vi "Update.vi"(10 "Value":dbl, 11 "OscillationDetector in":refnum<class "OscillationDetector.lvclass">) -> (3 "OscillationDetector out":refnum<class "OscillationDetector.lvclass">)   [LabVIEW 2019, in "OscillationDetector.lvclass"]
uses:
  OscillationDetector.lvclass
  OscillationDetector.lvclass/OscillationDetector.ctl
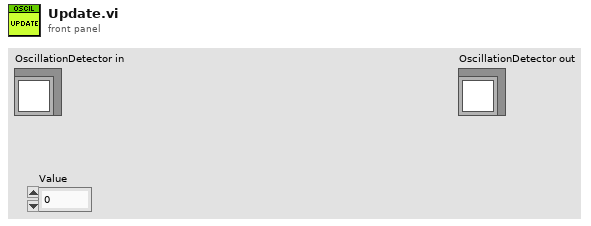
[diagram p1: front panel]
types:
  T1 = typedef "DATA Oscill.ctl" = cluster{"SUM":dbl, "COUNTER":dbl, "MAX CURR":dbl, "MIN CURR":dbl, "AVR":dbl, "MAX":dbl, "MIN":dbl, "DELTA AVR":dbl, "DELTA MAX":dbl, "DELTA MIN":dbl, "PERIOD":dbl}
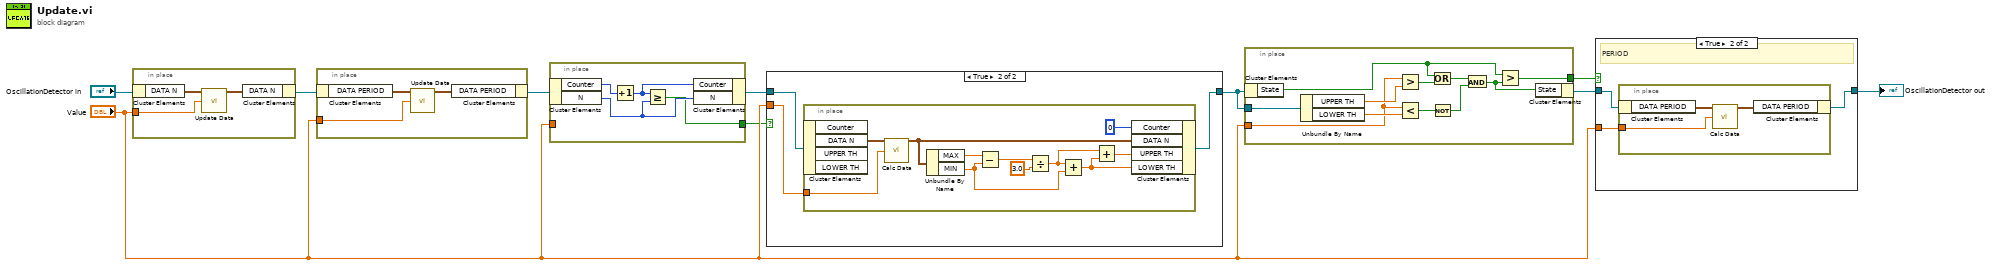
[diagram p0: block diagram]
diagram:
  n1 = in-place {
    in-place-border: "Value" -> [w11]
    n2 = in-place-cluster #1("OscillationDetector in") -> ("DATA N"=w13:T1)
    n3 = call "Update Data.vi"("DATA in"=w13, "Value"=w11) -> ("DATA iout"=w12:T1)  [unwired: 13 in]
    n4 = in-place-cluster #1("DATA N"=w12) -> (w9:refnum<class "OscillationDetector.lvclass">)
  }
  n5 = in-place {
    in-place-border: "Value" -> [w14]
    n6 = in-place-cluster #2(w9) -> ("DATA PERIOD"=w16:T1)
    n7 = call "Update Data.vi"("DATA in"=w16, "Value"=w14) -> ("DATA iout"=w15:T1)  [unwired: 13 in]
    n8 = in-place-cluster #2("DATA PERIOD"=w15) -> (w8:refnum<class "OscillationDetector.lvclass">)
  }
  n9 = in-place {
    in-place-border: "Value" -> [_]
    in-place-border: [w17] -> w4
    n10 = in-place-cluster #3(w8) -> ("Counter"=w20:i32, "N"=w18:i32)
    n11 = Increment(x=w20) -> (x+1=w19:i32)
    n12 = Greater Or Equal?(x=w19, y=w18) -> (x >= y?=w17:bool)
    n13 = in-place-cluster #3("Counter"=w19, "N"=w18) -> (w5:refnum<class "OscillationDetector.lvclass">)
  }
  n14 = case shown="True" w4 {
    tunnel: w5 -> [w21 w24]
    tunnel: [w21 w22] -> w3
    tunnel: "Value" -> [_ w23]
    frame False {
    }
    frame True {
      n15 = in-place {
        in-place-border: w23 -> [w34]
        n16 = in-place-cluster #4(w24) -> ("DATA N"=w35:T1)  [unwired: 3 out]
        n17 = call "Calc Data.vi"("DATA in"=w35, "Value"=w34) -> ("DATA iout"=w32:T1)  [unwired: 13 in]
        n18 = Unbundle By Name(w32) -> ("MAX"=w31:dbl, "MIN"=w28:dbl)
        n19 = Subtract(x=w31, y=w28) -> (x-y=w30:dbl)
        n20 = Divide(x=w30, y=3.0) -> (x/y=w26:dbl)
        n21 = Add(x=w26, y=w28) -> (x+y=w27:dbl)
        n22 = Add(x=w26, y=w27) -> (x+y=w25:dbl)
        n23 = in-place-cluster #4("Counter"=0, "DATA N"=w32, "UPPER TH"=w25, "LOWER TH"=w27) -> (w22:refnum<class "OscillationDetector.lvclass">)
      }
    }
  }
  n24 = in-place {
    in-place-border: w3 -> [w46]
    in-place-border: "Value" -> [w43]
    in-place-border: [w36] -> w1
    n25 = in-place-cluster #5(w3) -> ("State"=w38:bool)
    n26 = Unbundle By Name(w46) -> ("UPPER TH"=w45:dbl, "LOWER TH"=w44:dbl)
    n27 = Greater?(x=w43, y=w45) -> (0:w42:bool)
    n28 = Less?(x=w43, y=w44) -> (x < y?=w40:bool)
    n29 = Or(x=w38, y=w42) -> (x .or. y?=w41:bool)
    n30 = Not(x=w40) -> (.not. x?=w39:bool)
    n31 = And(x=w41, y=w39) -> (x .and. y?=w37:bool)
    n32 = Greater?(x=w38, y=w37) -> (0:w36:bool)
    n33 = in-place-cluster #5("State"=w37) -> (w7:refnum<class "OscillationDetector.lvclass">)
  }
  n34 = case shown="True" w1 {
    tunnel: w7 -> [w47 w50]
    tunnel: [w47 w49] -> w2
    tunnel: "Value" -> [_ w48]
    frame False {
    }
    frame True {
      # "PERIOD"
      n35 = in-place {
        in-place-border: w48 -> [w51]
        n36 = in-place-cluster #6(w50) -> ("DATA PERIOD"=w53:T1)
        n37 = call "Calc Data.vi"("DATA in"=w53, "Value"=w51) -> ("DATA iout"=w52:T1)  [unwired: 13 in]
        n38 = in-place-cluster #6("DATA PERIOD"=w52) -> (w49:refnum<class "OscillationDetector.lvclass">)
      }
    }
  }
  "OscillationDetector out" <- w2
